vi "distfc.vi"(0 "a":dbl, 5 "b":dbl, 7 "x":dbl, 9 "xv":dbl, 11 "yv":dbl) -> (4 "d":dbl, 8 "y-yv":dbl)   [LabVIEW 2015]
panel:
  out "yp":dbl
  out "y":dbl
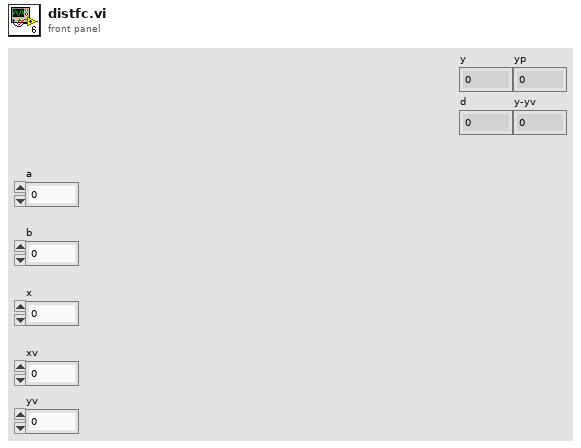
[diagram p1: front panel]
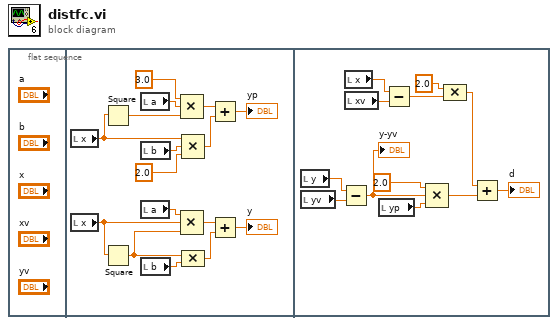
[diagram p0: block diagram]
diagram:
  n1 = flat-sequence {
    frame #0 {
    }
    frame #1 {
      n2 = local read "x"() -> (w3:dbl)
      n3 = local read "x"() -> (w15:dbl)
      n4 = Square(x=w3) -> (x^2=w4:dbl)
      n5 = Square(x=w15) -> (x^2=w14:dbl)
      n6 = local read "a"() -> (w6:dbl)
      n7 = local read "b"() -> (w7:dbl)
      n8 = local read "a"() -> (w16:dbl)
      n9 = local read "b"() -> (w13:dbl)
      n10 = Compound Arithmetic op=MULTIPLY(3.0 ("value"), w6, w4) -> (w8:dbl)
      n11 = Compound Arithmetic op=MULTIPLY(w16, w15, w14) -> (w12:dbl)
      n12 = Compound Arithmetic op=MULTIPLY(w3, w7, 2.0 ("value")) -> (w9:dbl)
      n13 = Compound Arithmetic op=MULTIPLY(w14, w13) -> (w11:dbl)
      n14 = Add(x=w8, y=w9) -> (x+y=→"yp":dbl)
      n15 = Add(x=w12, y=w11) -> (x+y=→"y":dbl)
    }
    frame #2 {
      n16 = local read "y"() -> (w23:dbl)
      n17 = local read "yv"() -> (w24:dbl)
      n18 = Subtract(x=w23, y=w24) -> (x-y=w18:dbl)
      "y-yv" <- w18
      n19 = local read "x"() -> (w27:dbl)
      n20 = local read "xv"() -> (w26:dbl)
      n21 = local read "yp"() -> (w21:dbl)
      n22 = Subtract(x=w27, y=w26) -> (x-y=w25:dbl)
      n23 = Compound Arithmetic op=MULTIPLY(2.0 ("value"), w18, w21) -> (w19:dbl)
      n24 = Compound Arithmetic op=MULTIPLY(2.0 ("value"), w25) -> (w20:dbl)
      n25 = Add(x=w20, y=w19) -> (x+y=→"d":dbl)
    }
  }
